vi "Wiimote Set Data Reporting.vi"(8 "error in":errorcluster, 9 "Reporting Mode":T1=48 items=["Status Information"=32, "Read Data"=33, "Write Data"=34, "Core Buttons"=48, "Core Buttons and Accelerometer"=49, "Core Buttons with 8 Extension bytes"=50, "Core Buttons and Accelerometer with 12 IR bytes"=51, "Core Buttons with 19 Extension bytes"=52, "Core Buttons and Accelerometer with 16 Extension Bytes"=53, "Core Buttons with 10 IR bytes and 9 Extension Bytes"=54, "Core Buttons and Accelerometer with 10 IR bytes and 6 Extension Bytes"=55], 10 "Continuous":bool, 11 "hWiimoteHandle in":u32 format="%08x") -> (0 "error out":errorcluster, 3 "hWiimoteHandle out":u32 format="%08x")   [LabVIEW 2011, in "Wiimote.lvlib"]
uses:
  Wiimote.lvlib
  Wiimote Reporting Mode.ctl
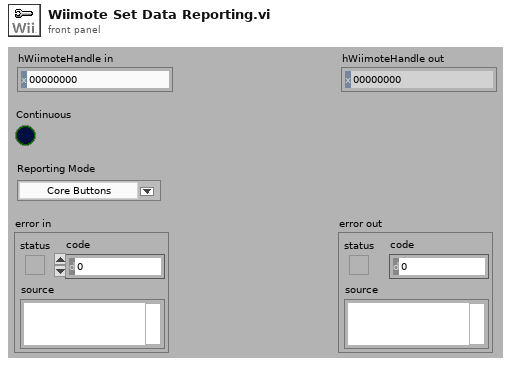
[diagram p1: front panel]
types:
  T1 = typedef "Wiimote.lvlib/Wiimote Reporting Mode.ctl" = u8
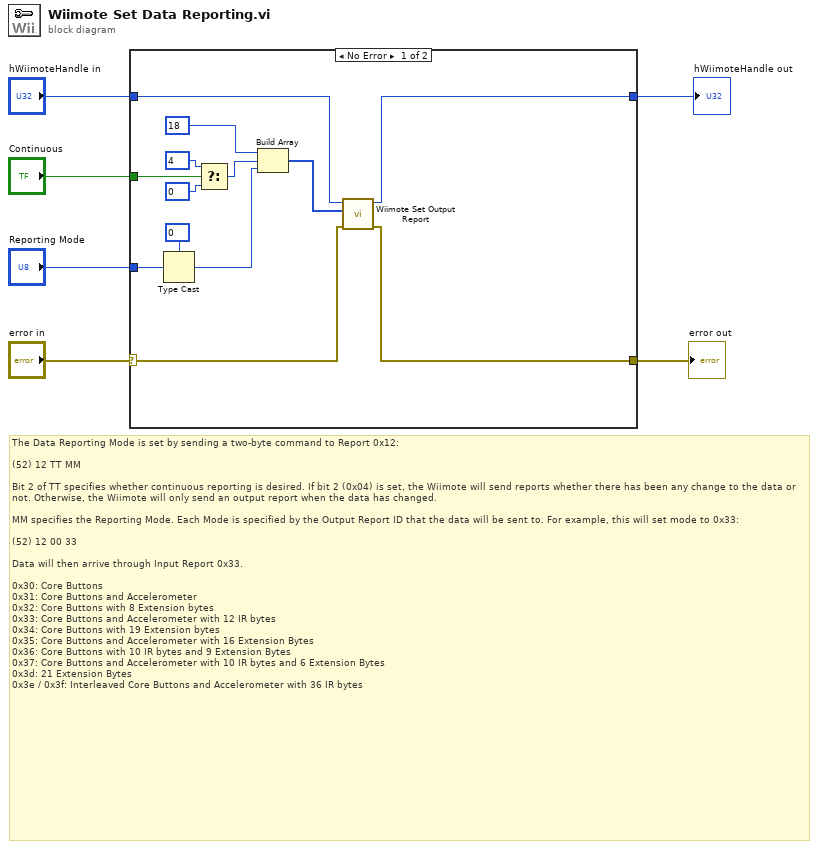
[diagram p0: block diagram]
diagram:
  # "The Data Reporting Mode is set by sending a two-byte command to Report 0x12:\n\n(52) 12 TT MM\n\nBit 2 of TT specifies whether continuous reporting is desired. If bit 2 (0x04) is set, the Wiimote will send reports whether there has been any change to the data or not. Otherwise, the Wiimote will only send an output report when the data has changed.\n\nMM specifies the Reporting Mode. Each Mode is specified by the Output Report ID that the data will be sent to. For example, this will set mode to 0x33:\n\n(52) 12 00 33\n\nData will then arrive through Input Report 0x33.\n\n0x30: Core Buttons\n0x31: Core Buttons and Accelerometer\n0x32: Core Buttons with 8 Extension bytes\n0x33: Core Buttons and Accelerometer with 12 IR bytes\n0x34: Core Buttons with 19 Extension bytes\n0x35: Core Buttons and Accelerometer with 16 Extension Bytes\n0x36: Core Buttons with 10 IR bytes and 9 Extension Bytes\n0x37: Core Buttons and Accelerometer with 10 IR bytes and 6 Extension Bytes\n0x3d: 21 Extension Bytes\n0x3e / 0x3f: Interleaved Core Buttons and Accelerometer with 36 IR bytes"
  n1 = case shown="No Error" "error in" {
    selector: "error in" -> [w8 w21]
    tunnel: [w7 w21] -> w5
    tunnel: "hWiimoteHandle in" -> [w13 w20]
    tunnel: [w12 w20] -> w3
    tunnel: "Reporting Mode" -> [w11 _]
    tunnel: "Continuous" -> [w14 _]
    frame No Error {
      n2 = Type Cast(type=u8 0, x=w11) -> (*(type *) &x=w9:u8)
      n3 = Select(t=u8 4, s=w14, f=u8 0) -> (s? t:f=w15:u8)
      n4 = Build Array(u8 18, w15, w9) -> (w18:u8[])
      n5 = call "Wiimote Set Output Report.vi"("error in"=w8, "pReportBuffer in"=w18, "hWiimoteHandle in"=w13) -> ("error out"=w7:errorcluster, "hWiimoteHandle out"=w12:u32)  [unwired: 7 in]
    }
    frame Error {
    }
  }
  "error out" <- w5
  "hWiimoteHandle out" <- w3
